vi "TCP-Com.vi"(8 "Exit Control Label":string="Exit Button", 9 "pwd":string, 10 "LabView Port":u16=4000, 11 "VI Refnum":refnum<vi>) -> (0 "error out":errorcluster)   [LabVIEW 2019]
doc: "This template is for the Queued Message Handler design pattern.\n\nThe Event Handling Loop generates messages based on user interface actions.\n\nThe Message Handling Loop processes messages generated by the Event Handling Loop, or by other messages. The messages are string values, so new messages can be added easily to the Message Cases case structure in the Message Handling Loop. Each message cluster can also provide an optional value for Message Data, which is a variant that can be converted to whatever message-specific data is required."
uses:
  support/TPC-Enum.ctl
  support/Message Queue/Enqueue Message (Single).vi
  support/Global 1.vi
  <vilib>/Utility/error.llb/Error Cluster From Error Code.vi
  <vilib>/ErrorRing/Error Ring.xnode
  support/Message Queue/Message Queue.lvlib
  support/User Event - Stop/User Event - Stop.lvlib
  <vilib>/Utility/Data Type/NI_Data Type.lvlib
panel:
  out "Sent to MIDAS":string
  out "connection ID":refnum<k5>
  out "Client Connected":bool
  in  "Request":string
  in  "Try request":bool
  in  "Exit":bool
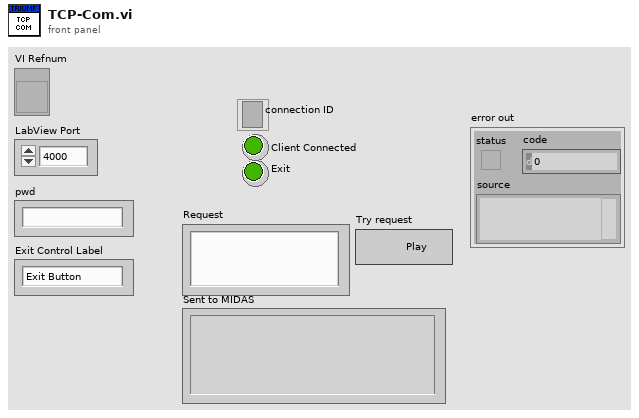
[diagram p1: front panel]
types:
  T1 = typedef "TPC-Enum.ctl" = enum16{"Wait For Client", "Check Client", "Listen"}
  T2 = typedef "Message Queue.lvlib/All Message Queues.ctl" = cluster{"TCP":refnum<queue>}
  T3 = typedef "NI_Data Type.lvlib/Data Type.ctl" = enum8{"Invalid Type", "Void", "I8", "I16", "I32", "I64", "U8", "U16", "U32", "U64", "Single Float", "Double Float", "Extended Float", "Single Complex", "Double Complex", "Extended Complex", "Enum U8", "Enum U16", "Enum U32", "Enum U64", "Single Float With Unit", "Double Float With Unit", "Extended Float With Unit", "Single Complex with Unit", "Double Complex with Unit", "Extended Complex with Unit", "Boolean", "String", "Path", "Picture", "Tag", "Array", "Cluster", "Variant", "LV Variant", "Waveform", "Timestamp", "Digital Waveform", "Digital Data", "ExpressData", "Refnum", "External Data", "VI", "Poly VI", "LabVIEW Class Instance", "Fixed Point", "Set Collection", "Map Collection"}
  T4 = enum16{"Standard", "Buffered", "CRLF", "Immediate"}
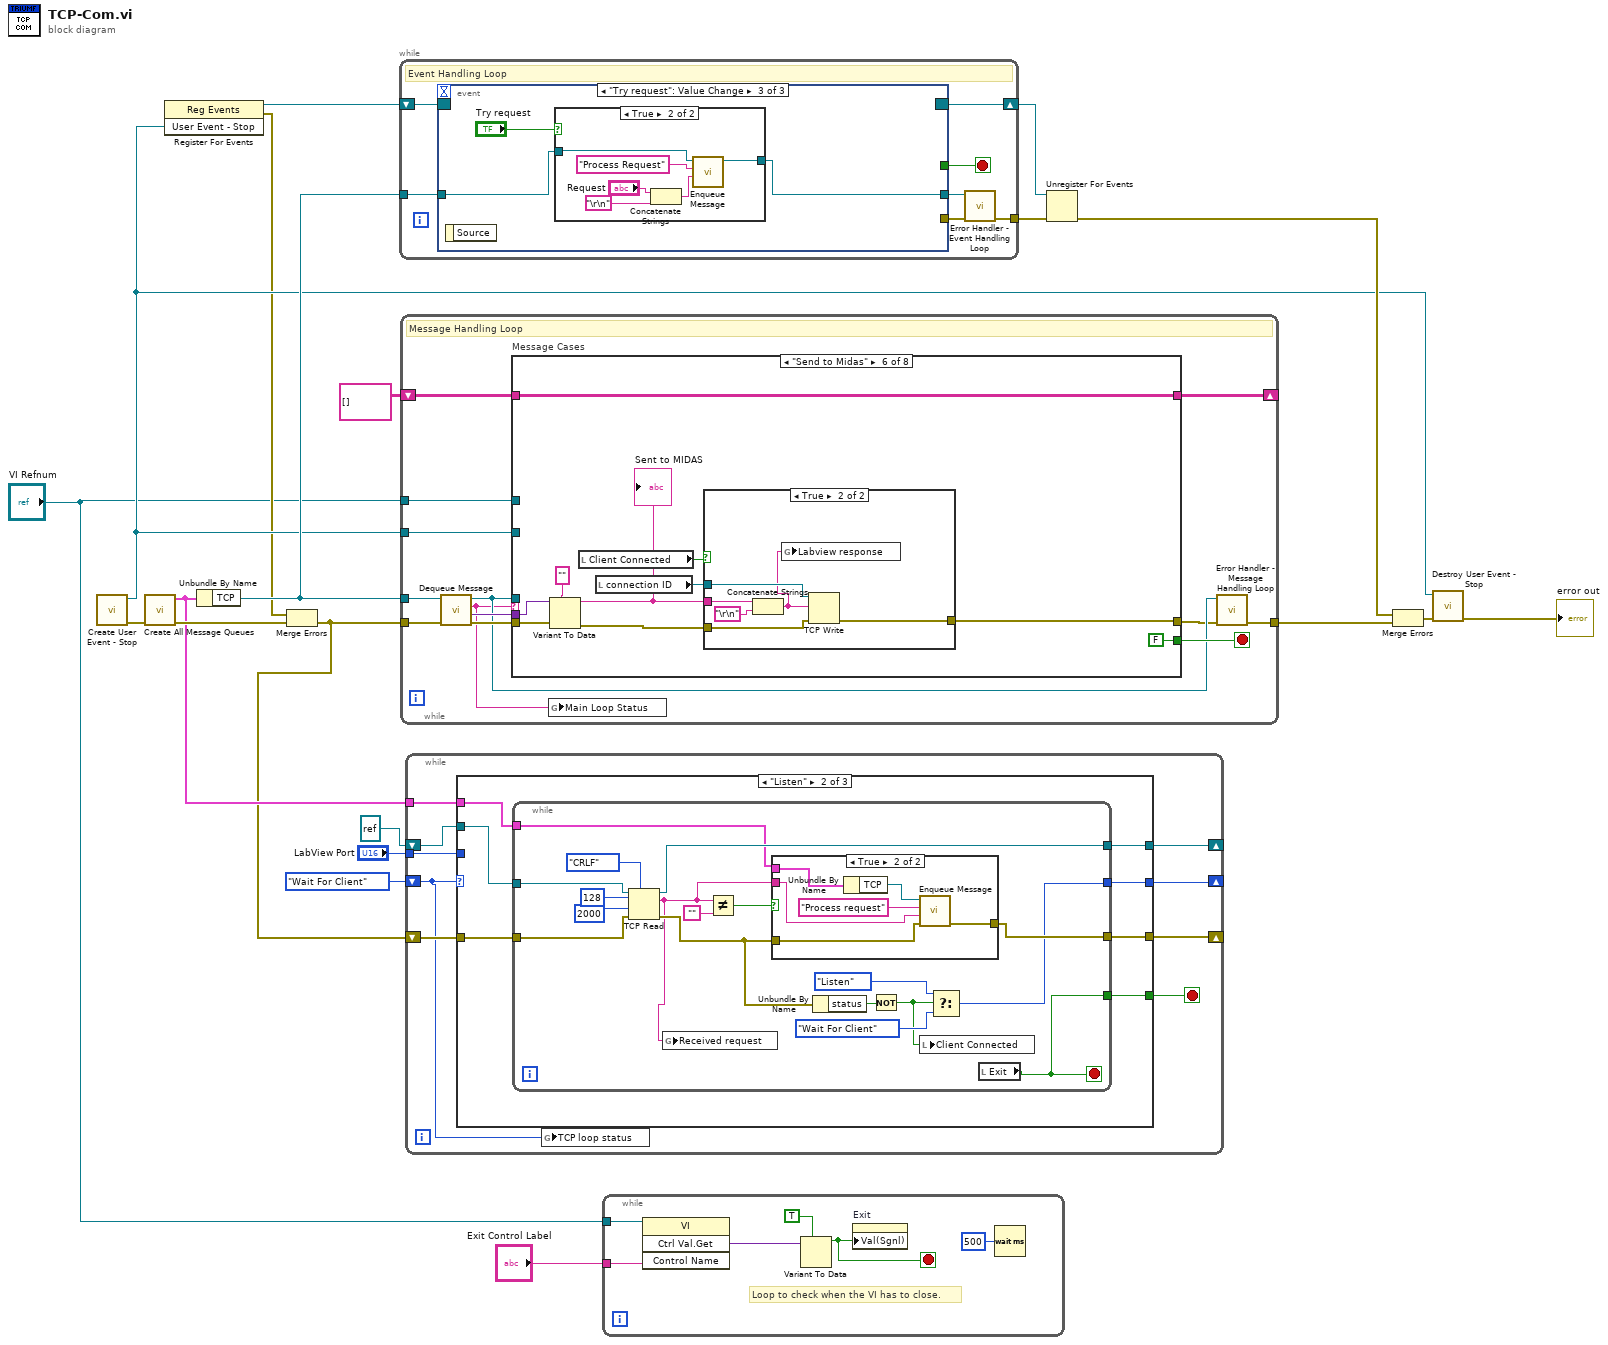
[diagram p0: block diagram]
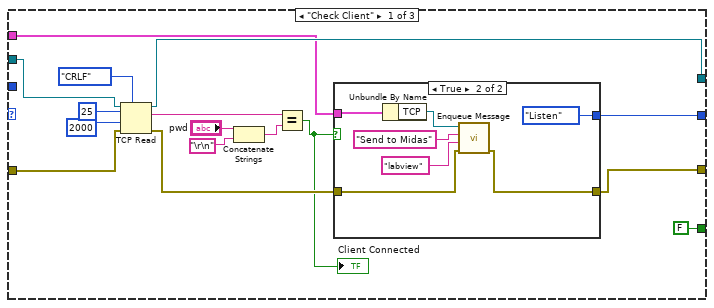
[diagram p2: hidden frame]
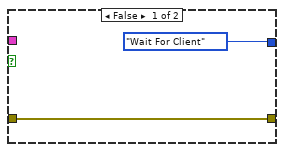
[diagram p3: hidden frame]
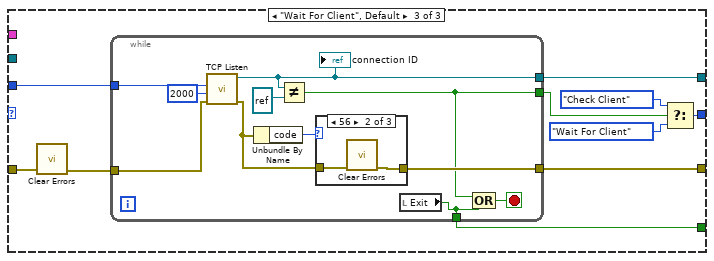
[diagram p5: hidden frame]
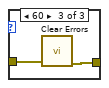
[diagram p7: hidden frame]
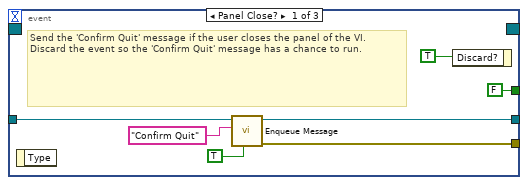
[diagram p8: hidden frame]
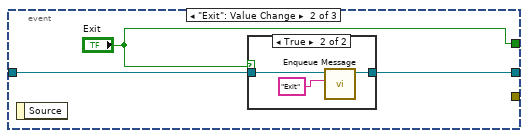
[diagram p9: hidden frame]
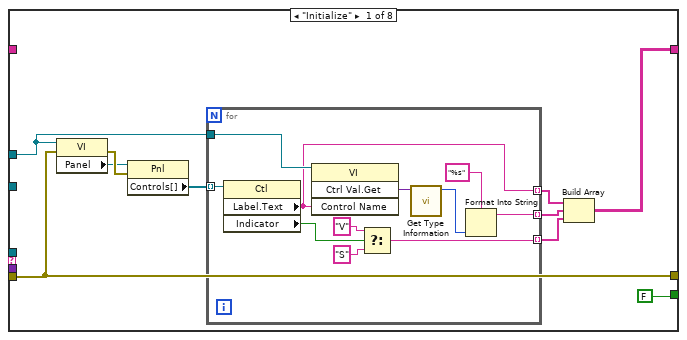
[diagram p12: hidden frame]
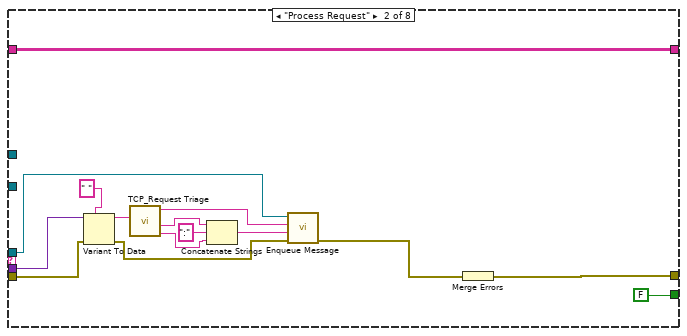
[diagram p13: hidden frame]
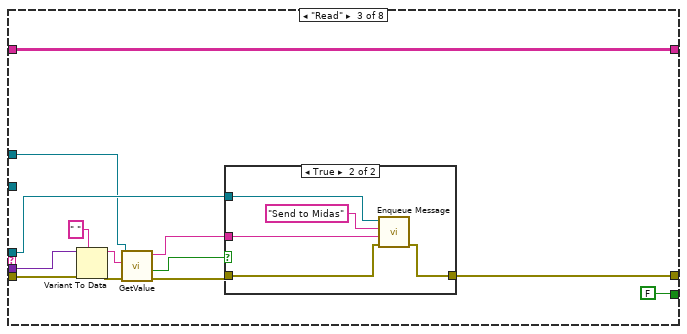
[diagram p14: hidden frame]
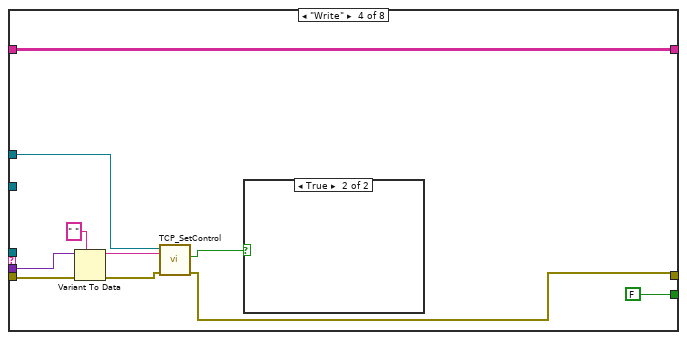
[diagram p16: hidden frame]
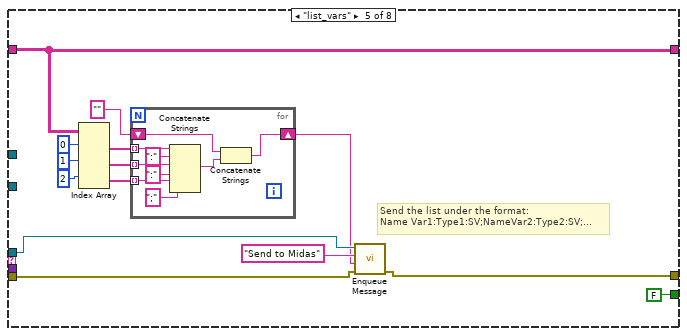
[diagram p18: hidden frame]
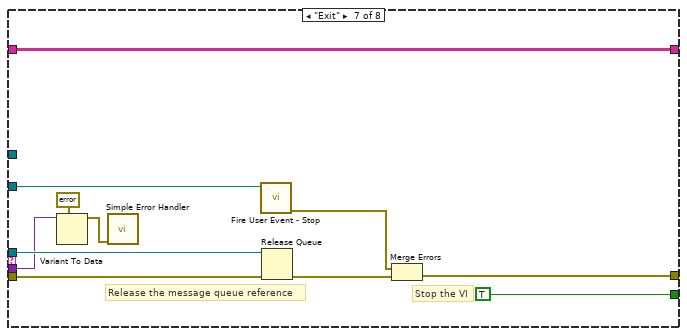
[diagram p20: hidden frame]
diagram:
  n1 = call "Create User Event - Stop.vi"() -> ("error out"=w17:errorcluster, "User Event - Stop"=w11:refnum<user-event>)  [unwired: 10 in]
  n2 = call "Create All Message Queues.vi"("error in (no error)"=w17) -> ("error out"=w20:errorcluster, "Message Queues out"=w6:T2)  [unwired: 9 in]
  n3 = register-events(w11) -> (reference out=w12:refnum<event-registration>, error out=w10:errorcluster)  [unwired: 2 in]
  n4 = Unbundle By Name(w6) -> ("TCP"=w18:refnum<queue>)
  n5 = Merge Errors(w10, w20) -> (w2:errorcluster)
  n6 = while {
    tunnel: w18 -> [w27]
    shift-right: [w25] -> w14
    shift-left: w12 -> [w26]
    tunnel: [w21] -> w13
    stop <- w23 stop-if-true
    # "Event Handling Loop"
    n7 = event shown="[2] \"Try request\": Value Change" {
      selector: w26 -> [_ _ _]
      dyn-events: [_ _ _] -> w25
      timeout: _ -> [_ _ _]
      tunnel: [FALSE ("Discard?") "Exit" _] -> w23
      tunnel: w27 -> [w33 w37 w43]
      tunnel: [w32 _ _] -> w24
      tunnel: [w31 w36 w42] -> w22
      event Panel Close? {
        # "Send the 'Confirm Quit' message if the user closes the panel of the VI. Discard the event so the 'Confirm Quit' message has a chance to run."
        n8 = event-data() -> ()  [unwired: 1 in, 1 out]
        n9 = call-poly "Enqueue Message.vi"("Priority Message? (F)"=TRUE, "Message"="Confirm Quit", "Message Queue"=w33) -> ("error out"=w32:errorcluster, "dup Message Queue"=w31:refnum<queue>)  [unwired: 7 in]
        n10 = event-data("Discard?"=TRUE) -> ()  [unwired: 1 in, 1 out]
      }
      event "Exit": Value Change {
        n11 = event-data() -> ()  [unwired: 1 in, 1 out]
        n12 = case shown="True" "Exit" {
          tunnel: w37 -> [w38 w41]
          tunnel: [w38 w39] -> w36
          frame False {
          }
          frame True {
            n13 = call-poly "Enqueue Message.vi"("Message"="Exit", "Message Queue"=w41) -> ("dup Message Queue"=w39:refnum<queue>)  [unwired: 8 in, 1 out]
          }
        }
      }
      event "Try request": Value Change {
        n14 = event-data() -> ()  [unwired: 1 in, 1 out]
        n15 = case shown="True" "Try request" {
          tunnel: w43 -> [w45 w50]
          tunnel: [w45 w49] -> w42
          frame False {
          }
          frame True {
            n16 = Concatenate Strings("Request", "\r\n") -> (w47:string)
            n17 = call-poly "Enqueue Message.vi"("Message Data"=w47, "Message"="Process Request", "Message Queue"=w50) -> ("dup Message Queue"=w49:refnum<queue>)  [unwired: 7 in, 1 out]
          }
        }
      }
    }
    n18 = call "Error Handler - Event Handling Loop.vi"("error in (no error)"=w24, "Message Queue"=w22) -> ("dup error in"=w21:errorcluster)  [unwired: 8 in, 1 out]
  }
  n19 = while {
    tunnel: w18 -> [w59]
    tunnel: w11 -> [w63]
    tunnel: w2 -> [w62]
    tunnel: [w57] -> w19
    tunnel: "VI Refnum" -> [w55]
    shift-right: [w54] -> _
    shift-left: string[][] [] -> [w53]
    stop <- w64 stop-if-true
    # "Message Handling Loop"
    n20 = call "Dequeue Message.vi"("error in (no error)"=w62, "Message Queue"=w59) -> ("error out"=w61:errorcluster, "Message Data"=w60:variant, "Message"=w52:string, "dup Message Queue"=w58:refnum<queue>)  [unwired: 6 in]
    n21 = case "Message Cases" shown="\"Send to Midas\"" w52 {
      selector: w52 -> [_ _ _ _ _ _ _ w183]
      tunnel: w58 -> [_ w93 w110 _ w142 _ w180 _]
      tunnel: w61 -> [w70 w98 w112 w128 w141 w160 w174 _]
      tunnel: [w70 w100 w109 w120 w140 w153 w177 w184] -> w56
      tunnel: [FALSE FALSE FALSE FALSE FALSE FALSE TRUE FALSE] -> w64
      tunnel: w60 -> [_ w99 w113 w127 _ w159 w171 _]
      tunnel: w63 -> [_ _ _ _ _ _ w176 _]
      tunnel: w55 -> [w69 _ w101 w123 _ _ _ _]
      tunnel: [w66 w86 w107 w125 w138 w162 w170 w181] -> w54
      tunnel: w53 -> [_ w86 w107 w125 w138 w162 w170 w181]
      frame "Initialize" {
        # "Initialize - All initialization work should take place in this message, since other loops can potentially enqueue messages that execute immediately after this one."
        n22 = property class="VI"(reference=w69, error in=w70) -> (error out=w73:errorcluster, "Panel"=w72:refnum<vi>)  [unwired: 1 out]
        n23 = property class="Pnl"(reference=w72, error in=w73) -> ("Controls[]"=w71:refnum<vi>[])  [unwired: 2 out]
        n24 = for {
          tunnel: w71 -> [w85] mode=indexing
          tunnel: w69 -> [w82]
          tunnel: [w80] -> w67 mode=indexing
          tunnel: [w79] -> w68 mode=indexing
          tunnel: [w75] -> w65 mode=indexing
          n25 = property class="Ctl"(reference=w85) -> ("Label.Text"=w79:string, "Indicator"=w78:bool)  [unwired: 1 in, 2 out]
          n26 = invoke class="VI" method="Ctrl Val.Get"(reference=w82, "Control Name"=w79) -> ("Get Control Value Variant"=w81:variant)  [unwired: 2 in, 3 out]
          n27 = Select(t="V" ("format string"), s=w78, f="S" ("format string")) -> (s? t:f=w75:string)
          n28 = call <vilib>:"Get Type Information.vi"("variant"=w81) -> ("type"=w83:T3)  [unwired: 6 in, 4 out]
          n29 = Format Into String(format string="%s", w83) -> (resulting string=w80:string)  [unwired: 2 in, 1 out]
        }
        n30 = Build Array(w68, w67, w65) -> (w66:string[][])
      }
      frame "Process Request" {
        # "Something - Replace this message with functionality for your own application."
        n31 = Variant To Data(error in=w98, type=" " ("Message"), Variant=w99) -> (data=w91:string, error out=w94:errorcluster)
        n32 = call "TCP_Request Triage.vi"("Message"=w91) -> ("Value"=w88:string, "Variable"=w89:string, "Request"=w90:string)  [unwired: 8 in]
        n33 = Concatenate Strings(w89, ":" ("string"), w88) -> (w92:string)
        n34 = call-poly "Enqueue Message.vi"("error in (no error)"=w94, "Message Data"=w92, "Message"=w90, "Message Queue"=w93) -> ("error out"=w95:errorcluster)  [unwired: 6 in, 1 out]
        n35 = Merge Errors(w95) -> (w100:errorcluster)
      }
      frame "Read" {
        n36 = Variant To Data(error in=w112, type=" " ("Message"), Variant=w113) -> (data=w102:string, error out=w106:errorcluster)
        n37 = call "GetValue.vi"("reference"=w101, "Input"=w102, "error in (no error)"=w106) -> ("Answer"=w104:string, "Found?"=w103:bool, "error out"=w105:errorcluster)  [unwired: 5 in]
        n38 = case shown="True" w103 {
          tunnel: [w114 w119] -> w109
          tunnel: w105 -> [w114 w118]
          tunnel: w110 -> [_ w117]
          tunnel: w104 -> [_ w115]
          frame False {
          }
          frame True {
            n39 = call-poly "Enqueue Message.vi"("error in (no error)"=w118, "Message Data"=w115, "Message"="Send to Midas", "Message Queue"=w117) -> ("error out"=w119:errorcluster)  [unwired: 6 in, 1 out]
          }
        }
      }
      frame "Write" {
        n40 = Variant To Data(error in=w128, type=" " ("Message"), Variant=w127) -> (data=w124:string, error out=w122:errorcluster)
        n41 = call "TCP_SetControl.vi"("VI Refnum"=w123, "Input"=w124, "error in (no error)"=w122) -> ("Found?"=w121:bool, "error out"=w120:errorcluster)  [unwired: 6 in]
        n42 = case shown="True" w121 {
          frame False {
          }
          frame True {
          }
        }
      }
      frame "list_vars" {
        # "Send the list under the format:\nName Var1:Type1:SV;NameVar2:Type2:SV;..."
        n43 = Index Array(array=w138, index (row) #1=0 ("index (row)"), index (row) #2=1 ("index (row)"), index (row) #3=2 ("index (row)")) -> (element #1=w136:string[], element #2=w134:string[], element #3=w130:string[])  [unwired: 3 in]
        n44 = for {
          tunnel: w136 -> [w152] mode=indexing
          tunnel: w134 -> [w150] mode=indexing
          shift-right: [w146] -> w132
          shift-left: "" -> [w148]
          tunnel: w130 -> [w145] mode=indexing
          n45 = Concatenate Strings(w152, ":" ("string"), w150, ":" ("string"), w145, ";" ("string")) -> (w147:string)
          n46 = Concatenate Strings(w148, w147) -> (w146:string)
        }
        n47 = call-poly "Enqueue Message.vi"("error in (no error)"=w141, "Message Data"=w132, "Message"="Send to Midas", "Message Queue"=w142) -> ("error out"=w140:errorcluster)  [unwired: 6 in, 1 out]
      }
      frame "Send to Midas" {
        n48 = Variant To Data(error in=w160, type="", Variant=w159) -> (data=w155:string, error out=w154:errorcluster)
        "Sent to MIDAS" <- w155
        n49 = local read "Client Connected"() -> (w157:bool)
        n50 = local read "connection ID"() -> (w156:refnum<k5>)
        n51 = case shown="True" w157 {
          tunnel: w156 -> [_ w166]
          tunnel: w155 -> [_ w169]
          tunnel: w154 -> [w163 w167]
          tunnel: [w163 w165] -> w153
          frame False {
          }
          frame True {
            n52 = Concatenate Strings(w169, "\r\n") -> (w164:string)
            n53 = global write "Global 1.vi" "Labview response"(w164) -> ()
            n54 = TCP Write(connection ID=w166, data in=w164, error in (no error)=w167) -> (error out=w165:errorcluster)  [unwired: 1 in, 2 out]
          }
        }
      }
      frame "Exit" {
        # "Stop the VI"
        # "Release the message queue reference"
        # "Exit - Exit the application."
        n55 = Variant To Data(type=errorcluster {"status"=FALSE, "code"=0, "source"=""} ("error constant"), Variant=w171) -> (data=w172:errorcluster)  [unwired: 1 in, 1 out]
        n56 = call <vilib>:"Simple Error Handler.vi"("error in (no error)"=w172) -> ()  [unwired: 4 in, 5 out]
        n57 = call "Fire User Event - Stop.vi"("User Event - Stop"=w176) -> ("error out"=w175:errorcluster)  [unwired: 10 in]
        n58 = Release Queue(queue=w180, error in (no error)=w174) -> (error out=w178:errorcluster)  [unwired: 1 in, 2 out]
        n59 = Merge Errors(w175, w178) -> (w177:errorcluster)
      }
      frame Default {
        # "'Default' case only runs if there is a message that isn't defined in any of the other cases.  Output a programming error."
        n60 = xnode "Error Ring"("parameter 0"=w183) -> ("error out"=w184:errorcluster)
      }
    }
    n61 = global write "Global 1.vi" "Main Loop Status"(w52) -> ()
    n62 = call "Error Handler - Message Handling Loop.vi"("error in (no error)"=w56, "Message Queue"=w58) -> ("dup error in"=w57:errorcluster)  [unwired: 8 in, 1 out]
  }
  n63 = while {
    shift-right: [w198] -> _
    shift-left: TPC-Enum."Wait For Client" -> [w192]
    tunnel: "LabView Port" -> [w200]
    shift-right: [w199] -> _
    shift-left: refnum<k5> refnum ("connection ID") -> [w194]
    shift-right: [w197] -> _
    shift-left: w2 -> [w196]
    tunnel: w6 -> [w193]
    stop <- w195 stop-if-true
    n64 = case shown="\"Listen\"" w192 {
      tunnel: w200 -> [_ _ w267]
      tunnel: w196 -> [w213 w231 w259]
      tunnel: [w207 w230 w266] -> w199
      tunnel: [w204 w227 w262] -> w198
      tunnel: [FALSE w226 w261] -> w195
      tunnel: [w203 w228 w260] -> w197
      tunnel: w194 -> [w212 w232 _]
      tunnel: w193 -> [w206 w229 _]
      frame "Check Client" {
        n65 = TCP Read(connection ID=w212, bytes to read=25, error in (no error)=w213, 7:T4."CRLF" ("mode (standard)"), 9:2000 ("timeout ms (25000)")) -> (connection ID out=w207:refnum<k5>, data out=w209:string, error out=w205:errorcluster)
        n66 = Concatenate Strings("pwd", "\r\n") -> (w208:string)
        n67 = Equal?(x=w209, y=w208) -> (x = y?=w201:bool)
        "Client Connected" <- w201
        n68 = case shown="True" w201 {
          tunnel: w206 -> [_ w225]
          tunnel: w205 -> [w218 w221]
          tunnel: [TPC-Enum."Wait For Client" TPC-Enum."Listen"] -> w204
          tunnel: [w218 w219] -> w203
          frame False {
          }
          frame True {
            n69 = Unbundle By Name(w225) -> ("TCP"=w224:refnum<queue>)
            n70 = call-poly "Enqueue Message.vi"("error in (no error)"=w221, "Message Data"="labview", "Message"="Send to Midas", "Message Queue"=w224) -> ("error out"=w219:errorcluster)  [unwired: 6 in, 1 out]
          }
        }
      }
      frame "Listen" {
        n71 = while {
          tunnel: w232 -> [w247]
          tunnel: w231 -> [w246]
          tunnel: [w243] -> w230
          tunnel: w229 -> [w242]
          tunnel: [w241] -> w228
          tunnel: [w236] -> w227
          tunnel: [w235] -> w226
          stop <- w235 stop-if-true
          n72 = TCP Read(connection ID=w247, bytes to read=128, error in (no error)=w246, 7:T4."CRLF" ("mode (standard)"), 9:2000 ("timeout ms (25000)")) -> (connection ID out=w243:refnum<k5>, data out=w233:string, error out=w239:errorcluster)
          n73 = global write "Global 1.vi" "Received request"(w233) -> ()
          n74 = Not Equal?(x=w233, y="") -> (x != y?=w244:bool)
          n75 = case shown="True" w244 {
            tunnel: w233 -> [_ w254]
            tunnel: w242 -> [_ w255]
            tunnel: w239 -> [w251 w253]
            tunnel: [w251 w252] -> w241
            frame False {
            }
            frame True {
              n76 = Unbundle By Name(w255) -> ("TCP"=w257:refnum<queue>)
              n77 = call-poly "Enqueue Message.vi"("error in (no error)"=w253, "Message Data"=w254, "Message"="Process request", "Message Queue"=w257) -> ("error out"=w252:errorcluster)  [unwired: 6 in, 1 out]
            }
          }
          n78 = Unbundle By Name(w239) -> ("status"=w240:bool)
          n79 = Not(x=w240) -> (.not. x?=w234:bool)
          n80 = local write "Client Connected"(w234) -> ()
          n81 = Select(t=TPC-Enum."Listen", s=w234, f=TPC-Enum."Wait For Client") -> (s? t:f=w236:T1)
          n82 = local read "Exit"() -> (w235:bool)
        }
      }
      frame "Wait For Client", Default {
        n83 = call <vilib>:"Clear Errors.vi"("error in (no error)"=w259) -> ("error out"=w258:errorcluster)  [unwired: 5 in, 1 out]
        n84 = while {
          tunnel: w267 -> [w278]
          tunnel: w258 -> [w276]
          tunnel: [w269] -> w265
          tunnel: [w274] -> w266
          tunnel: [w271] -> w260
          tunnel: [w268] -> w261
          stop <- w270 stop-if-true
          n85 = call <vilib>:"TCP Listen.vi"("error in (no error)"=w276, "timeout ms (wait forever: -1)"=2000, "port"=w278) -> ("error out"=w272:errorcluster, "connection ID"=w274:refnum<k5>)  [unwired: 4 in, 3 out]
          "connection ID" <- w274
          n86 = Unbundle By Name(w272) -> ("code"=w273:i32)
          n87 = Not Equal?(x=w274, y=refnum<k5> refnum ("connection ID")) -> (x != y?=w269:bool)
          n88 = case shown="56" w273 {
            tunnel: w272 -> [w279 w281 w283]
            tunnel: [w279 w280 w282] -> w271
            frame 0, Default {
            }
            frame 56 {
              n89 = call <vilib>:"Clear Errors.vi"("error in (no error)"=w281) -> ("error out"=w280:errorcluster)  [unwired: 5 in, 1 out]
            }
            frame 60 {
              n90 = call <vilib>:"Clear Errors.vi"("error in (no error)"=w283) -> ("error out"=w282:errorcluster)  [unwired: 5 in, 1 out]
            }
          }
          n91 = local read "Exit"() -> (w268:bool)
          n92 = Compound Arithmetic op=OR(w269, w268) -> (w270:bool)
        }
        n93 = Select(t=TPC-Enum."Check Client", s=w265, f=TPC-Enum."Wait For Client") -> (s? t:f=w262:T1)
      }
    }
    n94 = global write "Global 1.vi" "TCP loop status"(w192) -> ()
  }
  n95 = while {
    tunnel: "VI Refnum" -> [w284]
    tunnel: "Exit Control Label" -> [w285]
    stop <- w287 stop-if-true
    # "Loop to check when the VI has to close."
    n96 = invoke class="VI" method="Ctrl Val.Get"(reference=w284, "Control Name"=w285) -> ("Get Control Value Variant"=w286:variant)  [unwired: 2 in, 3 out]
    n97 = Variant To Data(type=TRUE, Variant=w286) -> (data=w287:bool)  [unwired: 1 in, 1 out]
    n98 = property on="Exit" class="Bool (strict)"("Val(Sgnl)"=w287) -> ()  [unwired: 2 in, 2 out]
    n99 = Wait (ms)(milliseconds to wait=u32 500) -> ()  [unwired: 1 out]
  }
  n100 = Unregister For Events(event registration refnum=w14, error in=w13) -> (error out=w15:errorcluster)
  n101 = Merge Errors(w15, w19) -> (w16:errorcluster)
  n102 = call "Destroy User Event - Stop.vi"("error in (no error)"=w16, "User Event - Stop"=w11) -> ("error out"=→"error out":errorcluster)  [unwired: 9 in]
